vi "LOEM_Lv_init.vi"(9 "Calibration Ch":i32(ring) items=["U00", "U01", "U02", "U03", "U04"], 10 "ManualMeasurementTime":dbl=0.1) -> (0 "error out":errorcluster, 3 "reference out":refnum<k24>)   [LabVIEW 2019]
uses:
  C:/Program Files (x86)/National Instruments/LabVIEW 2019/LC-MISDK.dll
  Program Files (x86)/National Instruments/LabVIEW 2019/LC-MISDK.dll
panel:
  # "Reprogramado Por Fredy Osorio 05/2025\ning.fredyosorio@gmail.com\nhttps://github.com/fr3dyos/PUC-LOEM-Controle-Minolta"
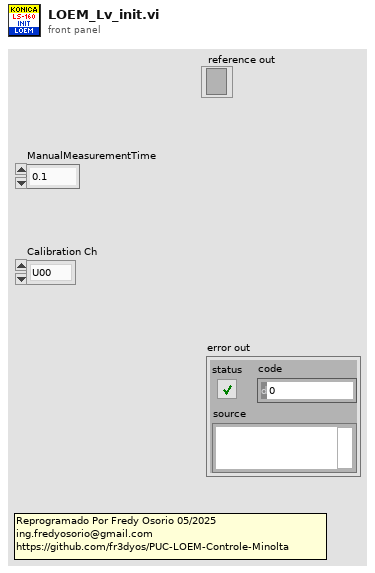
[diagram p1: front panel]
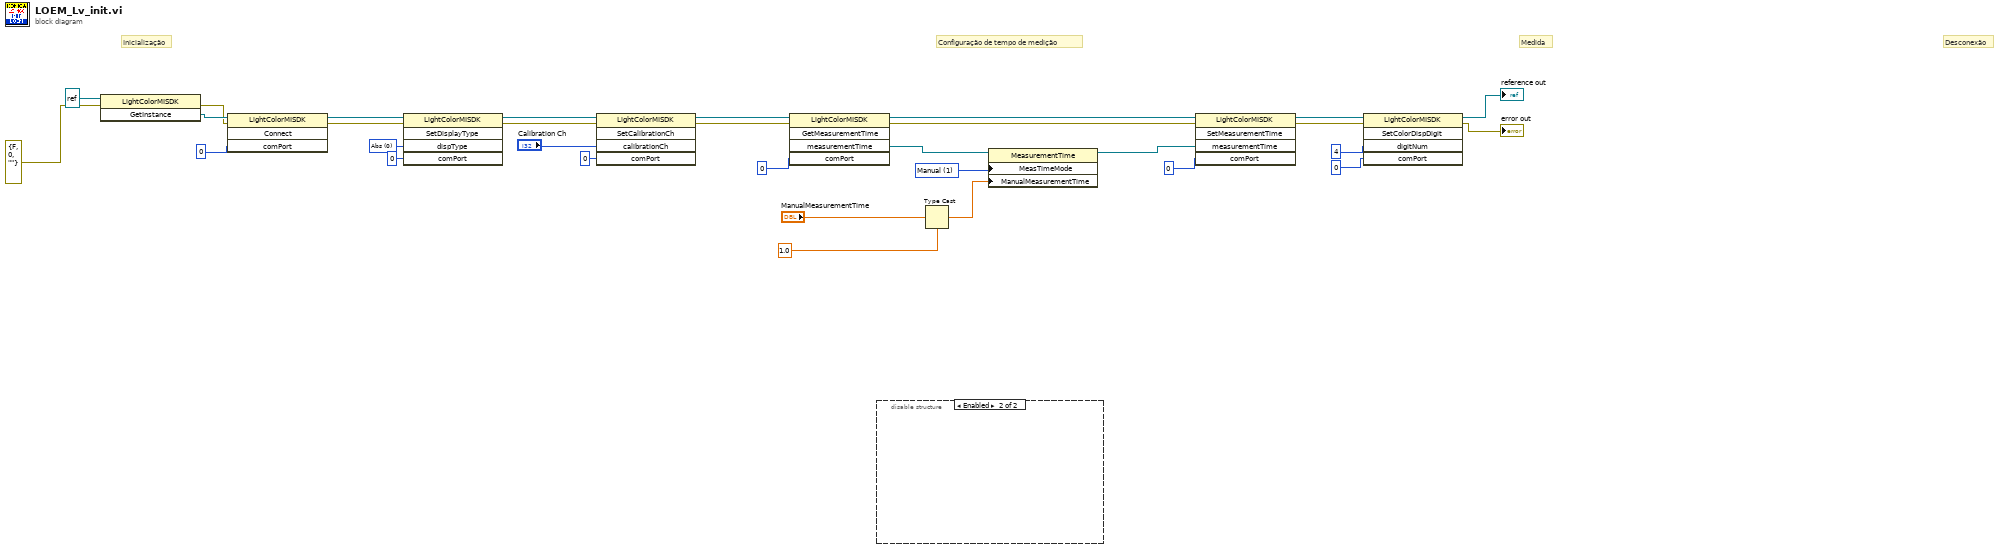
[diagram p0: block diagram]
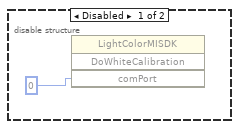
[diagram p2: hidden frame]
diagram:
  w14 = 0 items=["Abs", "Diff", "Ratio"] ("dispType")
  w28 = 1 items=["Auto", "Manual"] ("MeasTimeMode")
  # "Desconexão"
  # "Medida"
  # "Inicialização"
  # "Configuração de tempo de medição"
  n1 = invoke class="LightColorMISDK" method="GetInstance"(reference=refnum<k24> refnum, error in=errorcluster {"status"=FALSE, "code"=0, "source"=""} ("error in (no error)")) -> (error out=w8:errorcluster, "GetInstance"=w30:refnum<k24>)  [unwired: 1 in, 1 out]
  n2 = invoke class="LightColorMISDK" method="Connect"(reference=w30, error in=w8, "comPort"=0) -> (reference out=w16:refnum<k24>, error out=w7:errorcluster)  [unwired: 1 in, 2 out]
  n3 = invoke class="LightColorMISDK" method="SetDisplayType"(reference=w16, error in=w7, "dispType"=w14, "comPort"=0) -> (reference out=w13:refnum<k24>, error out=w6:errorcluster)  [unwired: 1 in, 3 out]
  n4 = invoke class="LightColorMISDK" method="SetCalibrationCh"(reference=w13, error in=w6, "calibrationCh"="Calibration Ch", "comPort"=0) -> (reference out=w12:refnum<k24>, error out=w5:errorcluster)  [unwired: 1 in, 3 out]
  n5 = invoke class="LightColorMISDK" method="GetMeasurementTime"(reference=w12, error in=w5, "comPort"=0) -> (reference out=w25:refnum<k24>, error out=w4:errorcluster, "measurementTime"=w24:refnum<k24>)  [unwired: 2 in, 2 out]
  n6 = disable-structure shown="Enabled" {
    frame Disabled {
      n7 = invoke class="LightColorMISDK" method="DoWhiteCalibration"("comPort"=0 ("DoWhiteCalibration")) -> ()  [unwired: 3 in, 4 out]
    }
    frame Enabled {
    }
  }
  n8 = Type Cast(type=1.0, x="ManualMeasurementTime") -> (*(type *) &x=w17:dbl)
  n9 = property class="MeasurementTime"(reference=w24, "MeasTimeMode"=w28, "ManualMeasurementTime"=w17) -> (reference out=w27:refnum<k24>)  [unwired: 1 in, 1 out]
  n10 = invoke class="LightColorMISDK" method="SetMeasurementTime"(reference=w25, error in=w4, "measurementTime"=w27, "comPort"=0) -> (reference out=w20:refnum<k24>, error out=w3:errorcluster)  [unwired: 1 in, 3 out]
  n11 = invoke class="LightColorMISDK" method="SetColorDispDigit"(reference=w20, error in=w3, "digitNum"=i16 4, "comPort"=0) -> (reference out=→"reference out":refnum<k24>, error out=→"error out":errorcluster)  [unwired: 1 in, 3 out]
